vi "CAN_LIN_FlexRay_AsynCall.vi"() -> ()   [LabVIEW 2014]
uses:
  <vilib>/Utility/miscctls.llb/LVPointTypeDef.ctl
  TypDef/CAN_LIN_FlexRay_Data.ctl
  CAN_LIN/TypDef/CAN_LIN_Data.ctl
panel:
  in  "CH_Mapping":bool
  in  "TS_Mapping":bool
  in  "Project_PATH":path=path "D:/Work/LabVIEW Code/TSMaster Labview SDK/LabVIEW/LabVIEW_TSMasterAPI_Demo_Old/TSMaster_FlexRay_Labview/TSMaster_FlexRay"
  in  "DLL_PATH":path=path "D:/Program Files (x86)/TOSUN/TSMaster/bin/TSMaster.dll"
  out "out put":T1={"Communication message"={"Sender"="", "receiver"="", "message"="", "data"=variant}, "Receive data"="", "error in"={"status"=FALSE, "code"=0, "source"=""}, "Data"={"DLL_PATH"=path "", "Call Array"=["CAN_Demo0", "LIN_Demo0"], "Project_PATH"=path ""}, "AsynCall?"=FALSE}
  in  "选项卡控件":enum32{"CAN", "LIN", "FlexRay"}(tab)
  in  "Config":bool
  in  "Connect":bool
  in  "Disconnect":bool
  out "Connect ?":bool
  in  "Creat error":bool
  in  "log":i32(listbox)
  in  "Quit":bool
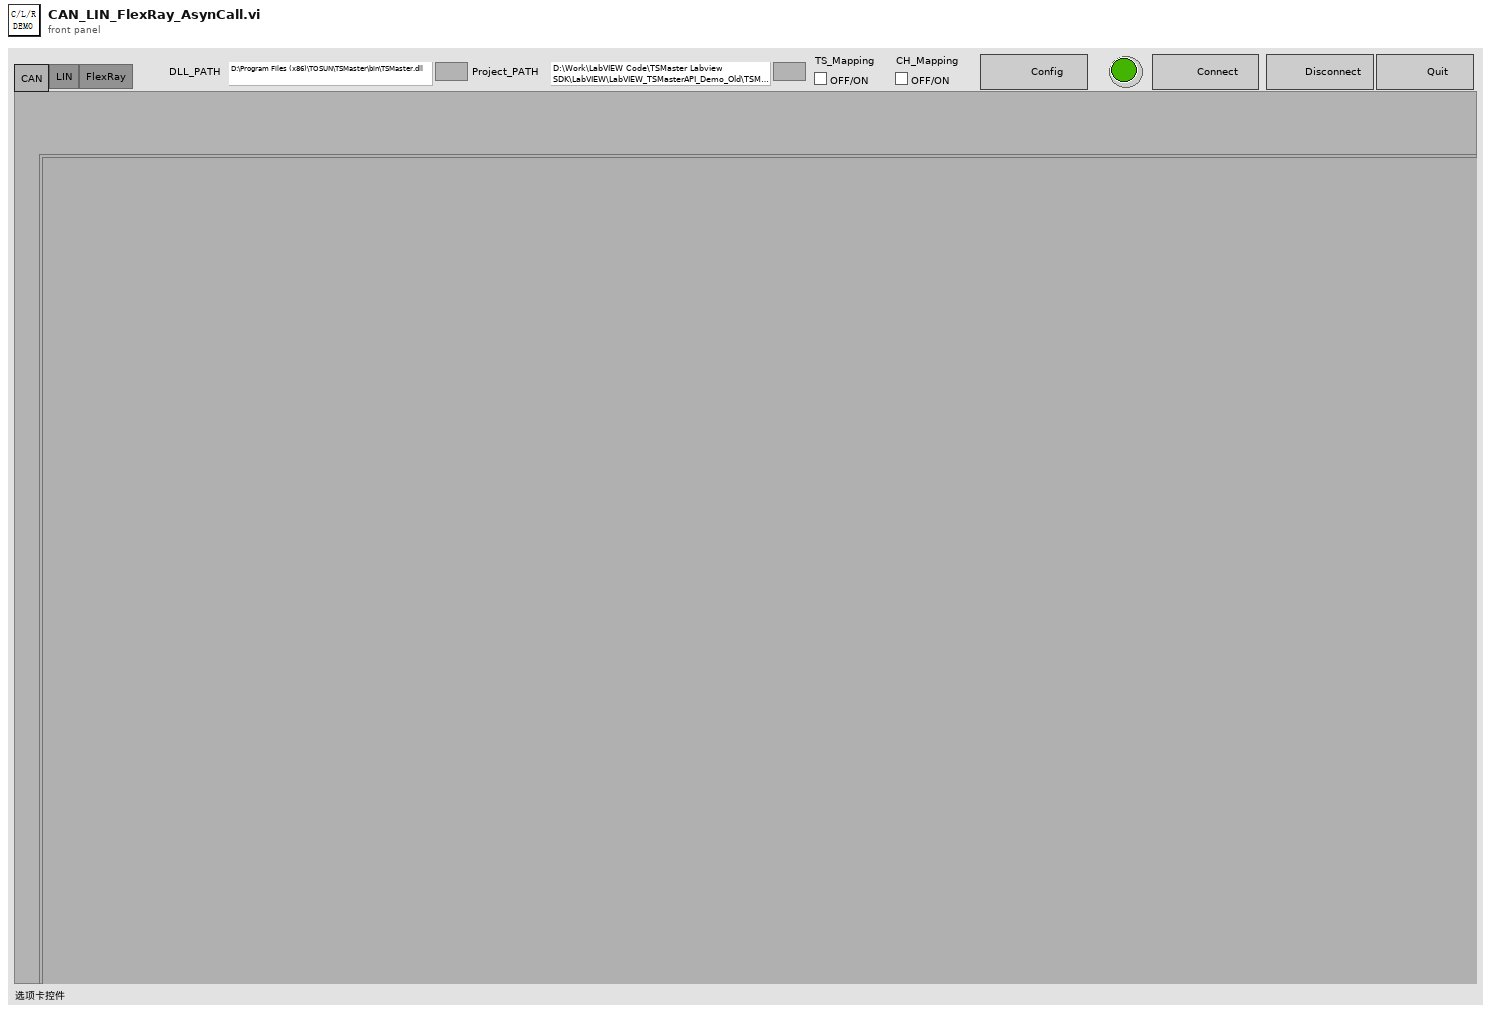
[diagram p1: front panel]
types:
  T1 = typedef "CAN_LIN_Data.ctl" = cluster{"Communication message":cluster{"Sender":string, "receiver":string, "message":string, "data":variant}, "Receive data":string, "error in":errorcluster, "Data":cluster{"DLL_PATH":path, "Call Array":string[], "Project_PATH":path}, "AsynCall?":bool}
  T2 = cluster{"Sender":string, "receiver":string, "message":string, "data":variant}
  T3 = typedef "CAN_LIN_FlexRay_Data.ctl" = cluster{"Communication message":cluster{"Sender":string, "receiver":string, "message":string, "data":variant}, "Receive data":string, "error in":errorcluster, "Data":cluster{"DLL_PATH":path, "Call Array":string[], "Project_PATH":path}, "AsynCall?":bool}
  T4 = typedef "LVPointTypeDef.ctl" = cluster{"Horizontal":i16, "Vertical":i16}
  T5 = enum32{"invalid app kind", "Development System", "Run Time System", "Student Edition", "Embedded LabVIEW", "Evaluation", "Custom"}
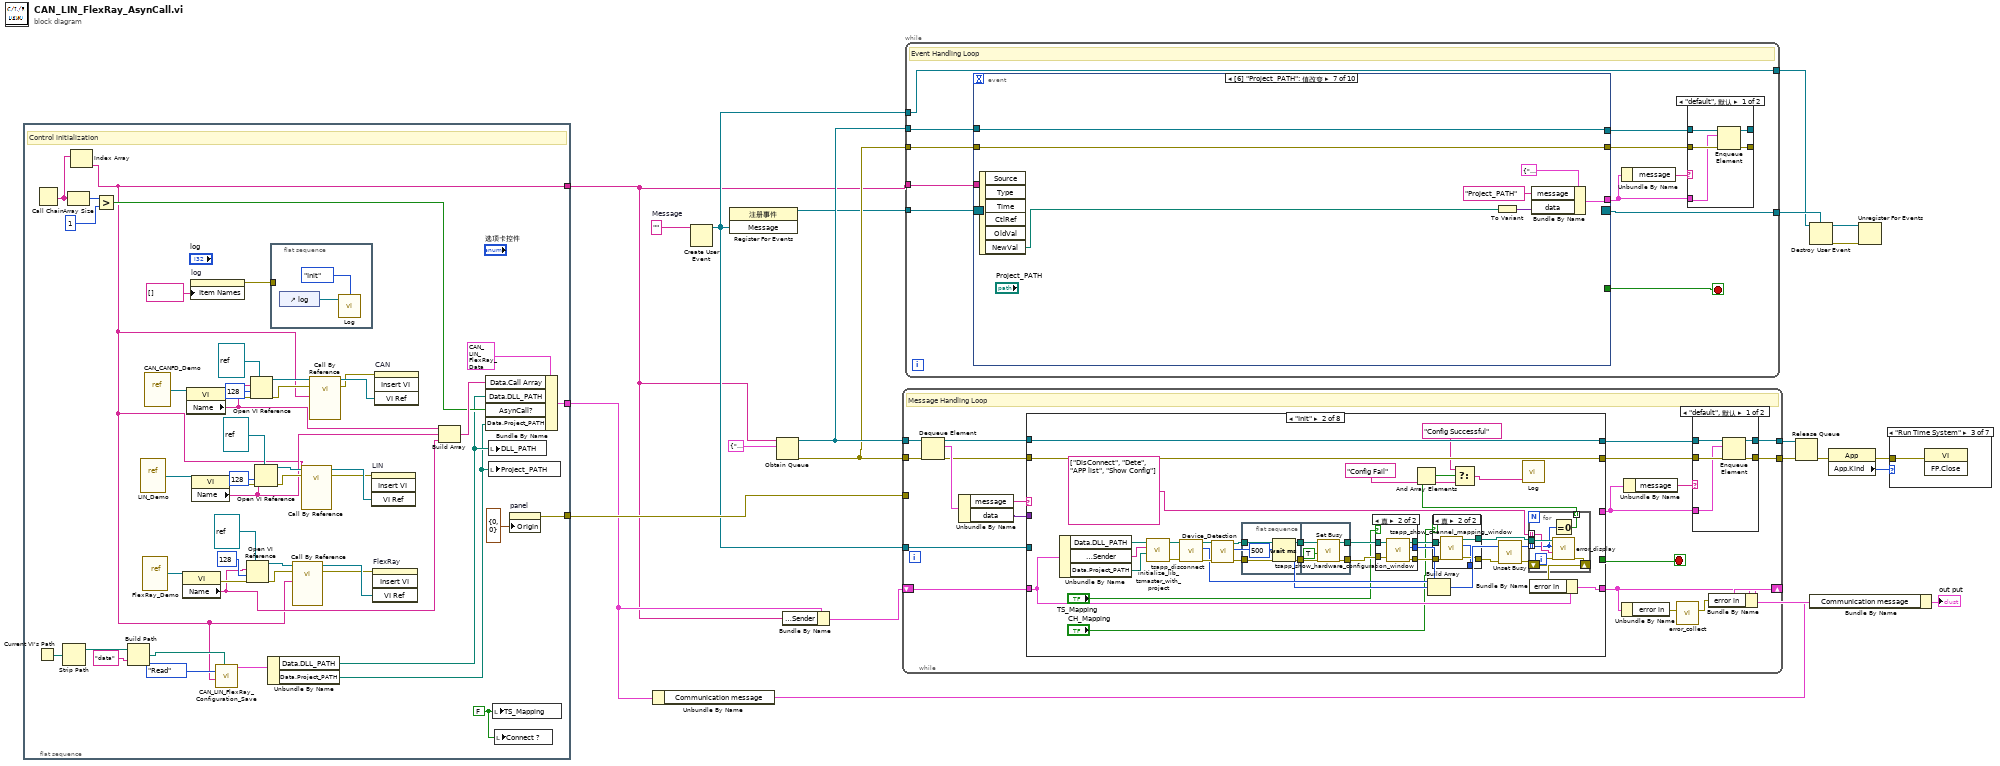
[diagram p0: block diagram]
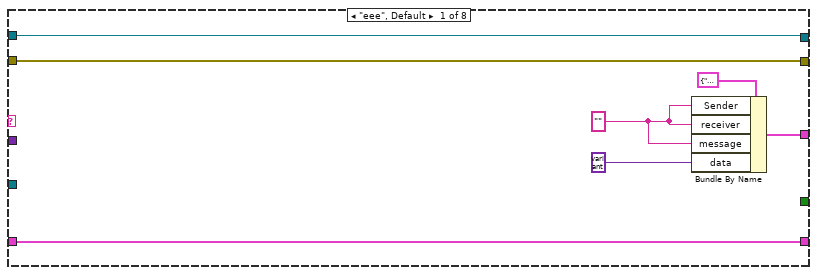
[diagram p9: hidden frame]
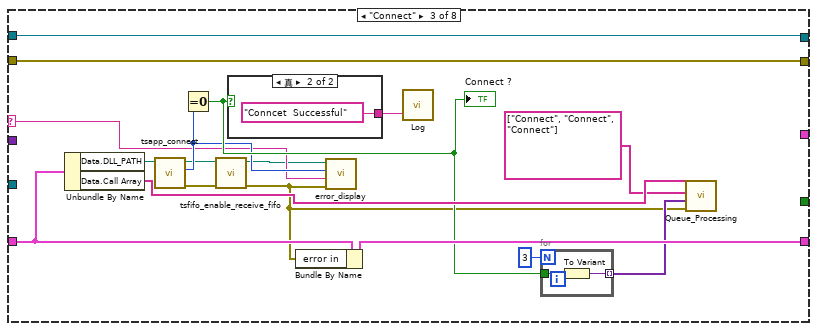
[diagram p12: hidden frame]
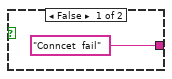
[diagram p13: hidden frame]
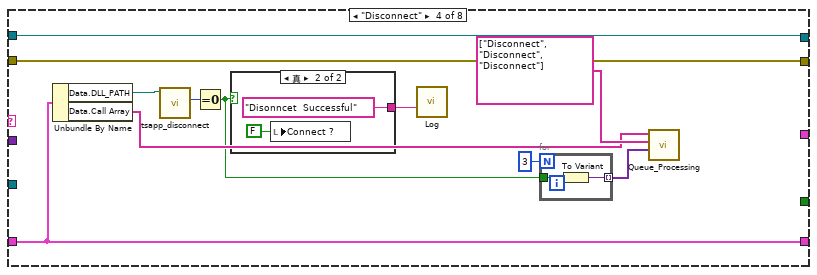
[diagram p14: hidden frame]
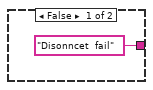
[diagram p15: hidden frame]
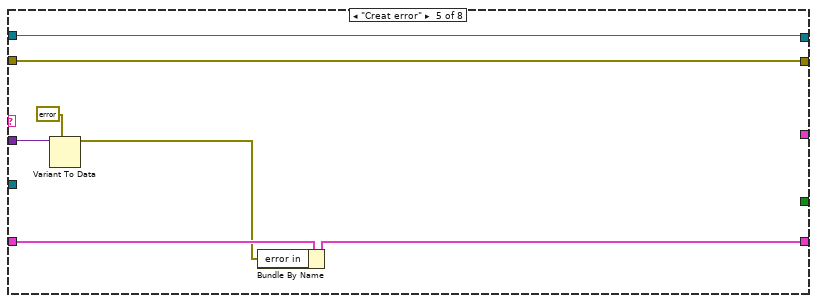
[diagram p16: hidden frame]
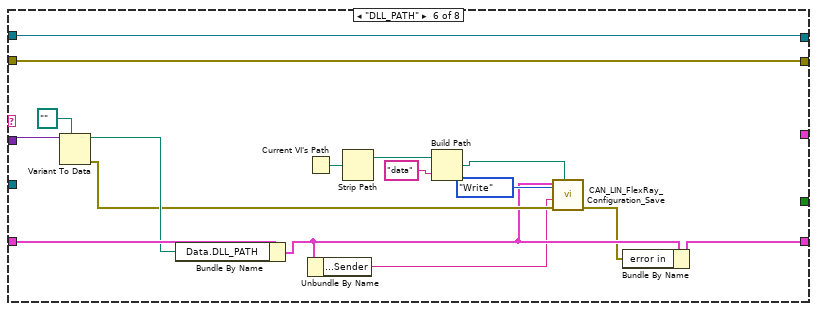
[diagram p17: hidden frame]
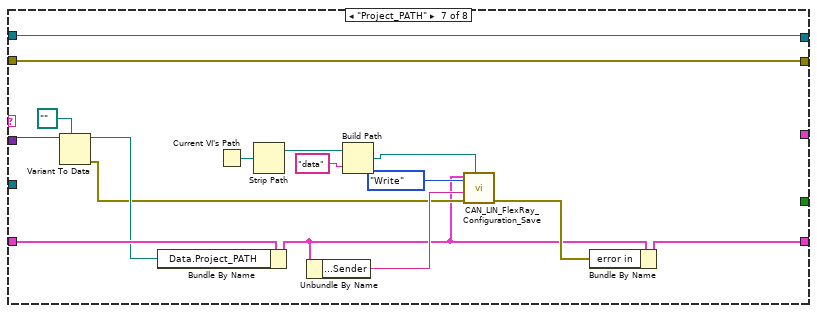
[diagram p18: hidden frame]
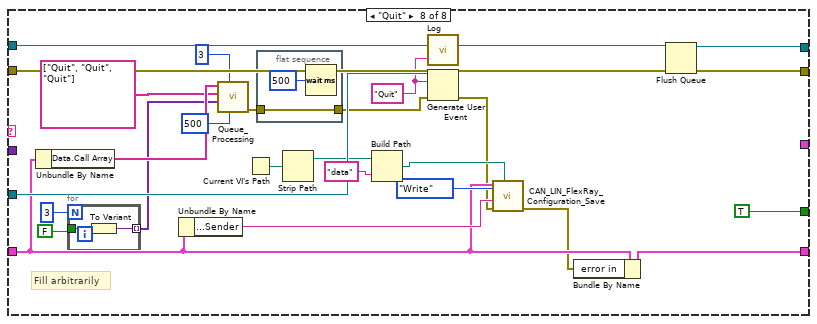
[diagram p19: hidden frame]
diagram:
  w12 = ""  # Message
  n1 = flat-sequence {
    tunnel: [w68] -> w10
    tunnel: [w49] -> w3
    tunnel: [w25] -> w1
    frame #0 {
      w32 = FALSE ("Connect ?")
      # "Control initialization"
      n2 = Current VI's Path() -> (path=w30:path)
      n3 = Call Chain() -> (call chain=w43:string[])
      n4 = Strip Path(path=w30) -> (stripped path=w28:path)  [unwired: 1 out]
      n5 = Array Size(array=w43) -> (size(s)=w45:i32)
      n6 = Index Array(array=w43) -> (element=w25:string)  [unwired: 1 in]
      n7 = Greater?(x=w45, y=1) -> (0:w42:bool)
      n8 = Build Path(base path=w28, name or relative path="data") -> (appended path=w27:path)
      n9 = vi-ref "LIN_Demo.vi"() -> (w65:refnum<vi>)
      n10 = vi-ref "FlexRay_Demo.vi"() -> (w36:refnum<vi>)
      n11 = vi-ref "CAN_CANFD_Demo.vi"() -> (w54:refnum<vi>)
      n12 = property class="VI"(reference=w36) -> (error out=w40:errorcluster, "Name"=w33:string)  [unwired: 1 in, 1 out]
      n13 = property class="VI"(reference=w54) -> (error out=w53:errorcluster, "Name"=w47:string)  [unwired: 1 in, 1 out]
      n14 = property on="log" class="LstBox (严格)"("Item Names"=string[] [] ("项名")) -> (error out=w66:errorcluster)  [unwired: 2 in, 1 out]
      n15 = property class="VI"(reference=w65) -> (error out=w52:errorcluster, "Name"=w46:string)  [unwired: 1 in, 1 out]
      n16 = call "CAN_LIN_FlexRay_Configuration_Save.vi"("path"=w27, "Config Name"=w25, "Read/Write"=enum16{"Read", "Write"}."Read") -> ("Data out"=w24:T3)  [unwired: 6 in, 2 out]
      n17 = Open VI Reference(type specifier VI Refnum (for type only)=refnum<vi> refnum ("类型说明符VI引用句柄（仅用于类型）"), vi path=w33, options=128 ("选项"), error in (no error)=w40) -> (vi reference=w38:refnum<vi>, error out=w39:errorcluster)  [unwired: 2 in]
      n18 = Open VI Reference(type specifier VI Refnum (for type only)=refnum<vi> refnum ("类型说明符VI引用句柄（仅用于类型）"), vi path=w47, options=128 ("选项"), error in (no error)=w53) -> (vi reference=w58:refnum<vi>, error out=w59:errorcluster)  [unwired: 2 in]
      n19 = Open VI Reference(type specifier VI Refnum (for type only)=refnum<vi> refnum ("类型说明符VI引用句柄（仅用于类型）"), vi path=w46, options=128 ("选项"), error in (no error)=w52) -> (vi reference=w63:refnum<vi>, error out=w60:errorcluster)  [unwired: 2 in]
      n20 = Unbundle By Name(w24) -> ("Data.DLL_PATH"=w23:path, "Data.Project_PATH"=w22:path)
      n21 = flat-sequence {
        tunnel: w66 -> [_]
        frame #0 {
          n22 = control-ref of="log"() -> (w70:refnum<vi>)
          n23 = call "Log.vi"("Method"=enum16{"Init", "Log"}."Init", "ListBox in"=w70) -> ()  [unwired: 2 in]
        }
      }
      n24 = call-by-ref "?"(reference=w38, error in=w39, "Sender"=w25) -> (reference out=w35:refnum<vi>, error out=w34:errorcluster)  [unwired: 11 in]
      n25 = call-by-ref "?"(reference=w63, error in=w60, "Sender"=w25) -> (reference out=w62:refnum<vi>, error out=w61:errorcluster)  [unwired: 11 in]
      n26 = call-by-ref "?"(reference=w58, error in=w59, "Sender"=w25) -> (reference out=w56:refnum<vi>, error out=w55:errorcluster)  [unwired: 11 in]
      n27 = invoke on="LIN" class="SubPnl" method="Insert VI"(error in=w61, "VI Ref"=w62) -> ()  [unwired: 2 in, 4 out]
      n28 = invoke on="FlexRay" class="SubPnl" method="Insert VI"(error in=w34, "VI Ref"=w35) -> ()  [unwired: 2 in, 4 out]
      n29 = invoke on="CAN" class="SubPnl" method="Insert VI"(error in=w55, "VI Ref"=w56) -> ()  [unwired: 2 in, 4 out]
      n30 = Build Array(w47, w46, w33) -> (w48:string[])
      n31 = Bundle By Name(cluster=T3 {"Communication message"={"Sender"="", "receiver"="", "message"="", "data"=variant}, "Receive data"="", "error in"={"status"=FALSE, "code"=0, "source"=""}, "Data"={"DLL_PATH"=path "", "Call Array"=["CAN_Demo0", "LIN_Demo0"], "Project_PATH"=path ""}, "AsynCall?"=FALSE} ("Data"), "Data.Call Array"=w48, "Data.DLL_PATH"=w23, "AsynCall?"=w42, "Data.Project_PATH"=w22) -> (w49:T3)
      n32 = local write "DLL_PATH"(w23) -> ()
      n33 = local write "Project_PATH"(w22) -> ()
      n34 = local write "TS_Mapping"(w32) -> ()
      n35 = local write "Connect ?"(w32) -> ()
      n36 = property on="panel" class="Pane"("Origin"=T4 {"Horizontal"=0, "Vertical"=0} ("原点")) -> (error out=w68:errorcluster)  [unwired: 2 in, 1 out]
    }
  }
  n37 = Unbundle By Name(w3) -> ("Communication message"=w4:T2)
  n38 = Create User Event(user event datatype=w12) -> (user event=w7:refnum<user-event>)  [unwired: 1 in, 1 out]
  n39 = register-events(w7) -> (reference out=w11:refnum<event-registration>)  [unwired: 2 in, 1 out]
  n40 = Obtain Queue(name (unnamed)=w1, element data type=T2 {"Sender"="", "receiver"="", "message"="", "data"=variant} ("Communication message")) -> (queue out=w21:refnum<queue>, error out=w14:errorcluster)  [unwired: 3 in, 1 out]
  n41 = Bundle By Name(cluster=w3, "Communication message.Sender"=w1) -> (w13:T3)
  n42 = while {
    tunnel: w21 -> [w91]
    tunnel: w14 -> [w90]
    tunnel: [w82] -> w20
    tunnel: [w81] -> w19
    shift-right: [w73] -> w5
    shift-left: w13 -> [w77]
    tunnel: w10 -> [_]
    tunnel: w7 -> [w76]
    stop <- w80 stop-if-true
    # "Message Handling Loop"
    n43 = Dequeue Element(queue=w91, error in (no error)=w90) -> (queue out=w87:refnum<queue>, element=w89:T2, error out=w86:errorcluster)  [unwired: 1 in, 1 out]
    n44 = Unbundle By Name(w89) -> ("message"=w88:string, "data"=w83:variant)
    n45 = case shown="\"Init\"" w88 {
      selector: w88 -> [_ _ w171 _ _ _ _ _]
      tunnel: [w105 w140 w184 w199 w211 w227 w243 w268] -> w85
      tunnel: w87 -> [w105 w140 w184 w199 w211 w227 w243 w267]
      tunnel: w86 -> [w104 w139 w183 w198 w210 w226 w242 w265]
      tunnel: [w104 w139 w183 w198 w210 w226 w242 w266] -> w84
      tunnel: w83 -> [_ _ _ _ w208 w224 w240 _]
      tunnel: [_ _ _ _ _ _ _ TRUE] -> w80
      tunnel: [w102 _ _ _ _ _ _ _] -> w79
      tunnel: [w99 w120 w179 w195 w206 w213 w230 w246] -> w75
      tunnel: w77 -> [w99 w121 w181 w195 w209 w225 w241 w248]
      tunnel: w76 -> [_ _ _ _ _ _ _ w264]
      frame "eee", Default {
        w100 = ""
        n46 = Bundle By Name(cluster=T2 {"Sender"="", "receiver"="", "message"="", "data"=variant} ("Communication message"), "Sender"=w100, "receiver"=w100, "message"=w100, "data"=variant) -> (w102:T2)
      }
      frame "Init" {
        n47 = Unbundle By Name(w121) -> ("Data.DLL_PATH"=w113:path, "Communication message.Sender"=w112:string, "Data.Project_PATH"=w136:path)
        n48 = call "initialize_lib_tsmaster_with_project.vi"("projectfile"=w136, "AppName"=w112, "Path input"=w113) -> ("error output"=w130:errorcluster, "Path output"=w132:path)  [unwired: 7 in]
        n49 = call "tsapp_disconnect.vi"("error in (no error)"=w130, "Path"=w132) -> ("error output"=w133:errorcluster, "retuen"=w129:i32, "Path output"=w131:path)  [unwired: 7 in]
        n50 = call "Device_Detection.vi"("error in (no error)"=w133, "Path"=w131) -> ("error out"=w123:errorcluster, "retuen"=w128:i32, "Path output"=w124:path)  [unwired: 7 in]
        n51 = flat-sequence {
          tunnel: w124 -> [w162]
          tunnel: w123 -> [w161]
          tunnel: [w162] -> w138
          tunnel: [w161] -> w137
          tunnel: [w165] -> w134
          tunnel: [w167] -> w135
          tunnel: w138 -> [w167]
          tunnel: w137 -> [w166]
          frame #0 {
            n52 = Wait (ms)(milliseconds to wait=u32 500) -> ()  [unwired: 1 out]
          }
          frame #1 {
            n53 = call <vilib>:"Set Busy.vi"("error in (no error)"=w166, "disable click? (T)"=TRUE) -> ("error out"=w165:errorcluster)  [unwired: 8 in, 1 out]
          }
        }
        n54 = case shown="真" "TS_Mapping" {
          tunnel: w135 -> [w149 w154]
          tunnel: w134 -> [w148 w153]
          tunnel: [w149 w152] -> w108
          tunnel: [_ w151] -> w126
          tunnel: [w148 w150] -> w110
          frame False {
          }
          frame True {
            n55 = call "tsapp_show_hardware_configuration_window.vi"("error in (no error)"=w153, "路径输入"=w154) -> ("error out"=w150:errorcluster, "function return"=w151:i32, "路径输出"=w152:path)  [unwired: 7 in]
          }
        }
        n56 = Build Array(w129, w128, w126) -> (w127:i32[])
        n57 = case shown="真" "CH_Mapping" {
          tunnel: w108 -> [w142 w147]
          tunnel: w110 -> [w141 w145]
          tunnel: [w142 w146] -> w107
          tunnel: [_ w143] -> _
          tunnel: [w141 w144] -> w109
          frame False {
          }
          frame True {
            n58 = call "tsapp_show_channel_mapping_window.vi"("error in (no error)"=w145, "路径输入"=w147) -> ("error out"=w144:errorcluster, "function return"=w143:i32, "路径输出"=w146:path)  [unwired: 7 in]
          }
        }
        n59 = call <vilib>:"Unset Busy.vi"("error in (no error)"=w109) -> ("error out"=w122:errorcluster)  [unwired: 10 in]
        n60 = for {
          tunnel: w107 -> [w158]
          shift-right: [w159] -> w119
          shift-left: w122 -> [w160]
          tunnel: w127 -> [w156] mode=indexing
          tunnel: string[] ["DisConnect", "Dete", "APP list", "Show Config"] -> [w157] mode=indexing
          tunnel: [w155] -> w115 mode=indexing
          n61 = Equal To 0?(x=w156) -> (x = 0?=w155:bool)
          n62 = call "error_display.vi"("error in"=w160, "Action name"=w157, "return"=w156, "DLL path"=w158) -> ("error out"=w159:errorcluster)  [unwired: 6 in, 1 out]
        }
        n63 = And Array Elements(Boolean array=w115) -> (logical AND=w118:bool)
        n64 = Select(t="Config Successful", s=w118, f="Config Fail") -> (s? t:f=w114:string)
        n65 = call "Log.vi"("Data"=w114) -> ()  [unwired: 3 in]
        n66 = Bundle By Name(cluster=w121, "error in"=w119) -> (w120:T3)
      }
      frame "Connect" {
        n67 = Unbundle By Name(w181) -> ("Data.DLL_PATH"=w180:path, "Data.Call Array"=w178:string[])
        n68 = call "tsapp_connect.vi"("Path"=w180) -> ("error out"=w169:errorcluster, "retuen"=w173:i32, "Path output"=w170:path)  [unwired: 8 in]
        n69 = Equal To 0?(x=w173) -> (x = 0?=w174:bool)
        "Connect ?" <- w174
        n70 = call "tsfifo_enable_receive_fifo.vi"("error in (no error)"=w169, "Path"=w170) -> ("error out"=w172:errorcluster, "Path output"=w168:path)  [unwired: 8 in]
        n71 = case shown="真" w174 {
          tunnel: ["Conncet  fail" ("消息") "Conncet  Successful" ("消息")] -> w182
          frame False {
          }
          frame True {
          }
        }
        n72 = Bundle By Name(cluster=w181, "error in"=w172) -> (w179:T3)
        n73 = call "error_display.vi"("error in"=w172, "Action name"=w171, "return"=w173, "DLL path"=w168) -> ()  [unwired: 6 in, 2 out]
        n74 = call "Log.vi"("Data"=w182) -> ()  [unwired: 3 in]
        n75 = for {
          N: 3 -> [_]
          tunnel: w174 -> [w186]
          tunnel: [w185] -> w176 mode=indexing
          n76 = To Variant(anything=w186) -> (Variant=w185:variant)
        }
        n77 = call "Queue_Processing.vi"("error in (no error)"=w172, "Data Array"=w176, "Cmd Array"=string[] ["Connect", "Connect", "Connect"], "Call Array"=w178) -> ()  [unwired: 7 in, 1 out]
      }
      frame "Disconnect" {
        n78 = Unbundle By Name(w195) -> ("Data.DLL_PATH"=w197:path, "Data.Call Array"=w190:string[])
        n79 = call "tsapp_disconnect.vi"("Path"=w197) -> ("retuen"=w194:i32)  [unwired: 8 in, 2 out]
        n80 = Equal To 0?(x=w194) -> (x = 0?=w189:bool)
        n81 = case shown="真" w189 {
          tunnel: ["Disonncet  fail" ("消息") "Disonncet  Successful" ("消息")] -> w196
          frame False {
          }
          frame True {
            n82 = local write "Connect ?"(FALSE ("Connect ?")) -> ()
          }
        }
        n83 = call "Log.vi"("Data"=w196) -> ()  [unwired: 3 in]
        n84 = for {
          N: 3 -> [_]
          tunnel: [w201] -> w192 mode=indexing
          tunnel: w189 -> [w200]
          n85 = To Variant(anything=w200) -> (Variant=w201:variant)
        }
        n86 = call "Queue_Processing.vi"("Data Array"=w192, "Cmd Array"=string[] ["Disconnect", "Disconnect", "Disconnect"], "Call Array"=w190) -> ()  [unwired: 8 in, 1 out]
      }
      frame "Creat error" {
        n87 = Variant To Data(type=errorcluster {"status"=FALSE, "code"=0, "source"=""} ("error out"), Variant=w208) -> (data=w205:errorcluster)  [unwired: 1 in, 1 out]
        n88 = Bundle By Name(cluster=w209, "error in"=w205) -> (w206:T3)
      }
      frame "DLL_PATH" {
        n89 = Variant To Data(type=path "" ("新值"), Variant=w224) -> (data=w222:path, error out=w216:errorcluster)  [unwired: 1 in]
        n90 = Bundle By Name(cluster=w225, "Data.DLL_PATH"=w222) -> (w215:T3)
        n91 = Current VI's Path() -> (path=w221:path)
        n92 = Unbundle By Name(w215) -> ("Communication message.Sender"=w214:string)
        n93 = Strip Path(path=w221) -> (stripped path=w219:path)  [unwired: 1 out]
        n94 = Build Path(base path=w219, name or relative path="data") -> (appended path=w218:path)
        n95 = call "CAN_LIN_FlexRay_Configuration_Save.vi"("path"=w218, "error in (no error)"=w216, "Config Name"=w214, "Read/Write"=enum16{"Read", "Write"}."Write", "Data"=w215) -> ("error in (no error)"=w212:errorcluster)  [unwired: 4 in, 2 out]
        n96 = Bundle By Name(cluster=w215, "error in"=w212) -> (w213:T3)
      }
      frame "Project_PATH" {
        n97 = Variant To Data(type=path "" ("新值"), Variant=w240) -> (data=w238:path, error out=w231:errorcluster)  [unwired: 1 in]
        n98 = Bundle By Name(cluster=w241, "Data.Project_PATH"=w238) -> (w228:T3)
        n99 = Current VI's Path() -> (path=w237:path)
        n100 = Strip Path(path=w237) -> (stripped path=w235:path)  [unwired: 1 out]
        n101 = Unbundle By Name(w228) -> ("Communication message.Sender"=w232:string)
        n102 = Build Path(base path=w235, name or relative path="data") -> (appended path=w234:path)
        n103 = call "CAN_LIN_FlexRay_Configuration_Save.vi"("path"=w234, "error in (no error)"=w231, "Config Name"=w232, "Read/Write"=enum16{"Read", "Write"}."Write", "Data"=w228) -> ("error in (no error)"=w229:errorcluster)  [unwired: 4 in, 2 out]
        n104 = Bundle By Name(cluster=w228, "error in"=w229) -> (w230:T3)
      }
      frame "Quit" {
        w263 = "Quit" ("y")
        # "Fill arbitrarily"
        n105 = Unbundle By Name(w248) -> ("Data.Call Array"=w260:string[])
        n106 = for {
          N: 3 -> [_]
          tunnel: [w271] -> w257 mode=indexing
          tunnel: FALSE -> [w270]
          n107 = To Variant(anything=w270) -> (Variant=w271:variant)
        }
        n108 = Unbundle By Name(w248) -> ("Communication message.Sender"=w249:string)
        n109 = call "Queue_Processing.vi"("Delay(ms)"=u32 500, "loop val"=3, "Data Array"=w257, "Cmd Array"=string[] ["Quit", "Quit", "Quit"], "Call Array"=w260) -> ("error out"=w262:errorcluster)  [unwired: 6 in]
        n110 = Current VI's Path() -> (path=w254:path)
        n111 = flat-sequence {
          tunnel: w262 -> [w272]
          tunnel: [w272] -> w261
          frame #0 {
            n112 = Wait (ms)(milliseconds to wait=u32 500 ("等待时间（毫秒）")) -> ()  [unwired: 1 out]
          }
        }
        n113 = Strip Path(path=w254) -> (stripped path=w252:path)  [unwired: 1 out]
        n114 = Build Path(base path=w252, name or relative path="data") -> (appended path=w251:path)
        n115 = call "Log.vi"("Data"=w263) -> ()  [unwired: 3 in]
        n116 = Generate User Event(user event=w264, event data cluster=w263, error in=w261) -> (error out=w247:errorcluster)  [unwired: 1 in, 1 out]
        n117 = call "CAN_LIN_FlexRay_Configuration_Save.vi"("path"=w251, "error in (no error)"=w247, "Config Name"=w249, "Read/Write"=enum16{"Read", "Write"}."Write", "Data"=w248) -> ("error in (no error)"=w245:errorcluster)  [unwired: 4 in, 2 out]
        n118 = Bundle By Name(cluster=w248, "error in"=w245) -> (w246:T3)
        n119 = Flush Queue(queue=w267, error in (no error)=w265) -> (queue out=w268:refnum<queue>, error out=w266:errorcluster)  [unwired: 1 out]
      }
    }
    n120 = Unbundle By Name(w75) -> ("error in"=w74:errorcluster)
    n121 = Unbundle By Name(w79) -> ("message"=w78:string)
    n122 = call "error_collect.vi"("error in (no error)"=w74) -> ("error IO"=w72:errorcluster)  [unwired: 10 in]
    n123 = case shown="\"default\", 默认" w78 {
      tunnel: w85 -> [w96 w98]
      tunnel: w84 -> [w95 w97]
      tunnel: w79 -> [w94 _]
      tunnel: [w93 w98] -> w82
      tunnel: [w92 w97] -> w81
      frame "default", Default {
        n124 = Enqueue Element(queue=w96, element=w94, error in (no error)=w95) -> (queue out=w93:refnum<queue>, error out=w92:errorcluster)  [unwired: 1 in, 1 out]
      }
      frame "" {
      }
    }
    n125 = Bundle By Name(cluster=w75, "error in"=w72) -> (w73:T3)
  }
  n126 = while {
    tunnel: w21 -> [w283]
    tunnel: w14 -> [w281]
    tunnel: w1 -> [w277]
    tunnel: w11 -> [w276]
    tunnel: [w275] -> w9
    tunnel: w7 -> [w274]
    tunnel: [w274] -> w6
    stop <- w284 stop-if-true
    # "Event Handling Loop"
    n127 = event shown="[6] \"Project_PATH\": 值改变" {
      selector: w276 -> [_ _ _ _ _ _ _ _ _ _]
      dyn-events: [_ _ _ _ _ _ _ _ _ _] -> w275
      timeout: _ -> [_ _ _ _ _ _ _ _ _ _]
      tunnel: [_ _ w301 w306 _ _ _ _ _ _] -> w284
      tunnel: w283 -> [w294 w299 w304 w309 w316 w323 w330 w335 w340 w345]
      tunnel: [w294 w299 w304 w307 w316 w323 w330 w335 w340 w345] -> w282
      tunnel: [T2 {"Sender"="", "receiver"="", "message"="", "data"=variant} ("Communication message") w297 _ _ w312 w319 w326 w331 w336 w341] -> w279
      tunnel: [w293 w295 w300 w305 w315 w322 w329 w334 w339 w344] -> w280
      tunnel: w281 -> [w293 w295 w300 w305 w315 w322 w329 w334 w339 w344]
      tunnel: w277 -> [_ _ _ _ _ _ _ _ _ _]
      event Timeout {
        n128 = event-data() -> ()  [unwired: 1 in, 3 out]
      }
      event "Quit": Value Change {
        n129 = event-data() -> ()  [unwired: 1 in, 6 out]
        n130 = Bundle By Name(cluster=T2 {"Sender"="", "receiver"="", "message"="", "data"=variant} ("Communication message"), "message"="Quit" ("Sender")) -> (w297:T2)
      }
      event User Event {
        n131 = event-data() -> ("Message"=w303:string)  [unwired: 1 in]
        n132 = Equal?(x=w303, y="Quit") -> (x = y?=w301:bool)
      }
      event Panel Close? {
        w306 = TRUE ("放弃？")
        n133 = event-data() -> ()  [unwired: 1 in, 4 out]
        n134 = Enqueue Element(queue=w309, element=T2 {"Sender"="", "receiver"="", "message"="Quit", "data"=variant} ("Communication message")) -> (queue out=w307:refnum<queue>)  [unwired: 2 in, 2 out]
        n135 = event-data("Discard?"=w306) -> ()  [unwired: 1 in, 1 out]
      }
      event "Creat error": Value Change {
        n136 = event-data() -> ()  [unwired: 1 in, 6 out]
        n137 = To Variant(anything=errorcluster {"status"=TRUE, "code"=709394, "source"="This is a error demo"}) -> (Variant=w310:variant)
        n138 = Bundle By Name(cluster=T2 {"Sender"="", "receiver"="", "message"="", "data"=variant} ("Communication message"), "message"="Creat error" ("Sender"), "data"=w310) -> (w312:T2)
      }
      event "DLL_PATH": Value Change {
        n139 = event-data() -> ("NewVal"=w317:path)  [unwired: 1 in, 5 out]
        n140 = To Variant(anything=w317) -> (Variant=w318:variant)
        n141 = Bundle By Name(cluster=T2 {"Sender"="", "receiver"="", "message"="", "data"=variant} ("Communication message"), "message"="DLL_PATH" ("Sender"), "data"=w318) -> (w319:T2)
      }
      event "Project_PATH": Value Change {
        n142 = event-data() -> ("NewVal"=w324:path)  [unwired: 1 in, 5 out]
        n143 = To Variant(anything=w324) -> (Variant=w325:variant)
        n144 = Bundle By Name(cluster=T2 {"Sender"="", "receiver"="", "message"="", "data"=variant} ("Communication message"), "message"="Project_PATH" ("Sender"), "data"=w325) -> (w326:T2)
      }
      event "Config": Value Change {
        n145 = event-data() -> ()  [unwired: 1 in, 6 out]
        n146 = Bundle By Name(cluster=T2 {"Sender"="", "receiver"="", "message"="", "data"=variant} ("Communication message"), "message"="Init" ("Sender")) -> (w331:T2)
      }
      event "Connect": Value Change {
        n147 = event-data() -> ()  [unwired: 1 in, 6 out]
        n148 = Bundle By Name(cluster=T2 {"Sender"="", "receiver"="", "message"="", "data"=variant} ("Communication message"), "message"="Connect" ("Sender")) -> (w336:T2)
      }
      event "Disconnect": Value Change {
        n149 = event-data() -> ()  [unwired: 1 in, 6 out]
        n150 = Bundle By Name(cluster=T2 {"Sender"="", "receiver"="", "message"="", "data"=variant} ("Communication message"), "message"="Disconnect" ("Sender")) -> (w341:T2)
      }
    }
    n151 = Unbundle By Name(w279) -> ("message"=w278:string)
    n152 = case shown="\"default\", 默认" w278 {
      tunnel: w282 -> [w289 w291]
      tunnel: w280 -> [w288 w290]
      tunnel: w279 -> [w287 _]
      tunnel: [w286 w291] -> _
      tunnel: [w285 w290] -> _
      frame "default", Default {
        n153 = Enqueue Element(queue=w289, element=w287, error in (no error)=w288) -> (queue out=w286:refnum<queue>, error out=w285:errorcluster)  [unwired: 1 in, 1 out]
      }
      frame "" {
      }
    }
  }
  n154 = Release Queue(queue=w20, error in (no error)=w19) -> (error out=w18:errorcluster)  [unwired: 1 in, 2 out]
  n155 = Destroy User Event(user event=w6) -> (error out=w8:errorcluster)  [unwired: 1 in]
  n156 = Bundle By Name(cluster=w5, "Communication message"=w4) -> (→"out put":T3)
  n157 = property class="App"(error in=w18) -> (error out=w17:errorcluster, "App.Kind"=w16:T5)  [unwired: 1 in, 1 out]
  n158 = Unregister For Events(event registration refnum=w9, error in=w8) -> ()  [unwired: 1 out]
  n159 = case shown="\"Run Time System\"" w16 {
    tunnel: w17 -> [_ _ w346 _ _ _ _]
    frame "invalid app kind", Default {
    }
    frame "Development System" {
    }
    frame "Run Time System" {
      n160 = invoke class="VI" method="FP.Close"(error in=w346) -> ()  [unwired: 2 in, 3 out]
    }
    frame "Student Edition" {
    }
    frame "Embedded LabVIEW" {
    }
    frame "Evaluation" {
    }
    frame "Custom" {
    }
  }
